vi "Settings.vi"(0 "error in":errorcluster, 1 "Channel A Settings":T2={"Enabled"=FALSE, "Coupling"=1, "Range"=6, "Analogue Offset"=0.0} {"Range" items=["10 mV", "20 mV", "50 mV", "100 mV", "200 mV", "500 mV", "1 V", "2 V", "5 V", "10 V", "20 V"]; "Coupling" items=["AC", "DC"]}, 2 "Port 0 Settings":cluster{"Enabled":bool, "Logic Level":i16}={"Enabled"=FALSE, "Logic Level"=9830} {"Logic Level" items=["1.5V TTL"=9830, "2.5V CMOS"=16383]}, 3 "Channel B Settings":T2={"Enabled"=FALSE, "Coupling"=1, "Range"=6, "Analogue Offset"=0.0} {"Range" items=["10 mV", "20 mV", "50 mV", "100 mV", "200 mV", "500 mV", "1 V", "2 V", "5 V", "10 V", "20 V"]; "Coupling" items=["AC", "DC"]}, 5 "handle in":i16, 9 "Device Info":T1, 11 "Trigger Settings":T3={"Trigger Enabled"=FALSE, "Trigger Source"=enum."Channel A", "Trigger Threshold (volts)"=0.0, "Trigger Direction"=2, "Trigger Delay (samples)"=0, "Auto Trigger Time (ms)"=1000} {"Trigger Direction" items=["Rising"=2, "Falling"=3]}, 12 "Channel C Settings":T2={"Enabled"=FALSE, "Coupling"=1, "Range"=6, "Analogue Offset"=0.0} {"Range" items=["10 mV", "20 mV", "50 mV", "100 mV", "200 mV", "500 mV", "1 V", "2 V", "5 V", "10 V", "20 V"]; "Coupling" items=["AC", "DC"]}, 13 "Port 1 Settings":cluster{"Enabled":bool, "Logic Level":i16}={"Enabled"=FALSE, "Logic Level"=9830} {"Logic Level" items=["1.5V TTL"=9830, "2.5V CMOS"=16383]}, 14 "Channel D Settings":T2={"Enabled"=FALSE, "Coupling"=1, "Range"=6, "Analogue Offset"=0.0} {"Range" items=["10 mV", "20 mV", "50 mV", "100 mV", "200 mV", "500 mV", "1 V", "2 V", "5 V", "10 V", "20 V"]; "Coupling" items=["AC", "DC"]}, 15 "Max ADC value":i16) -> (4 "error out":errorcluster, 6 "handle out":i16, 8 "enabled array":i16[](array[numeric]))   [LabVIEW 2017]
doc: "This VI is used to set up the oscilloscope. The inputs are clusters for setting channel and simple trigger settings. Advanced triggers can be set up using PicoScope3000aAdvancedTriggerSettings.vi"
uses:
  ps5000a.dll
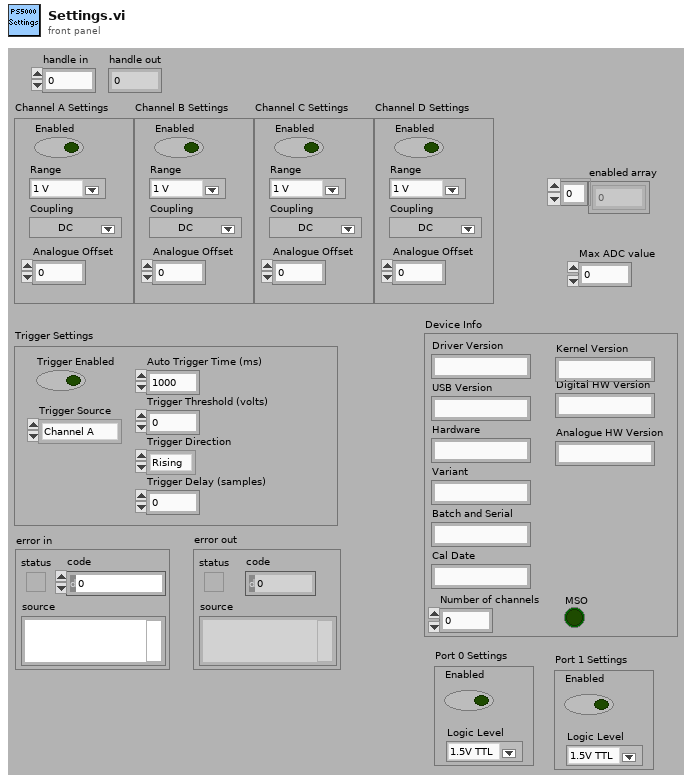
[diagram p1: front panel]
types:
  T1 = cluster{"Driver Version":string, "USB Version":string, "Hardware":string, "Variant":string, "Batch and Serial":string, "Cal Date":string, "Kernel Version":string, "Digital HW Version":string, "Analogue HW Version":string, "MSO":bool, "Number of channels":i16}
  T2 = cluster{"Enabled":bool, "Coupling":i16, "Range":u16, "Analogue Offset":sgl}
  T3 = cluster{"Trigger Enabled":bool, "Trigger Source":enum16{"Channel A", "Channel B", "Channel C", "Channel D", "Ext."}, "Trigger Threshold (volts)":dbl, "Trigger Direction":u16, "Trigger Delay (samples)":u32, "Auto Trigger Time (ms)":i16}
  T4 = enum16{"Channel A", "Channel B", "Channel C", "Channel D", "Ext."}
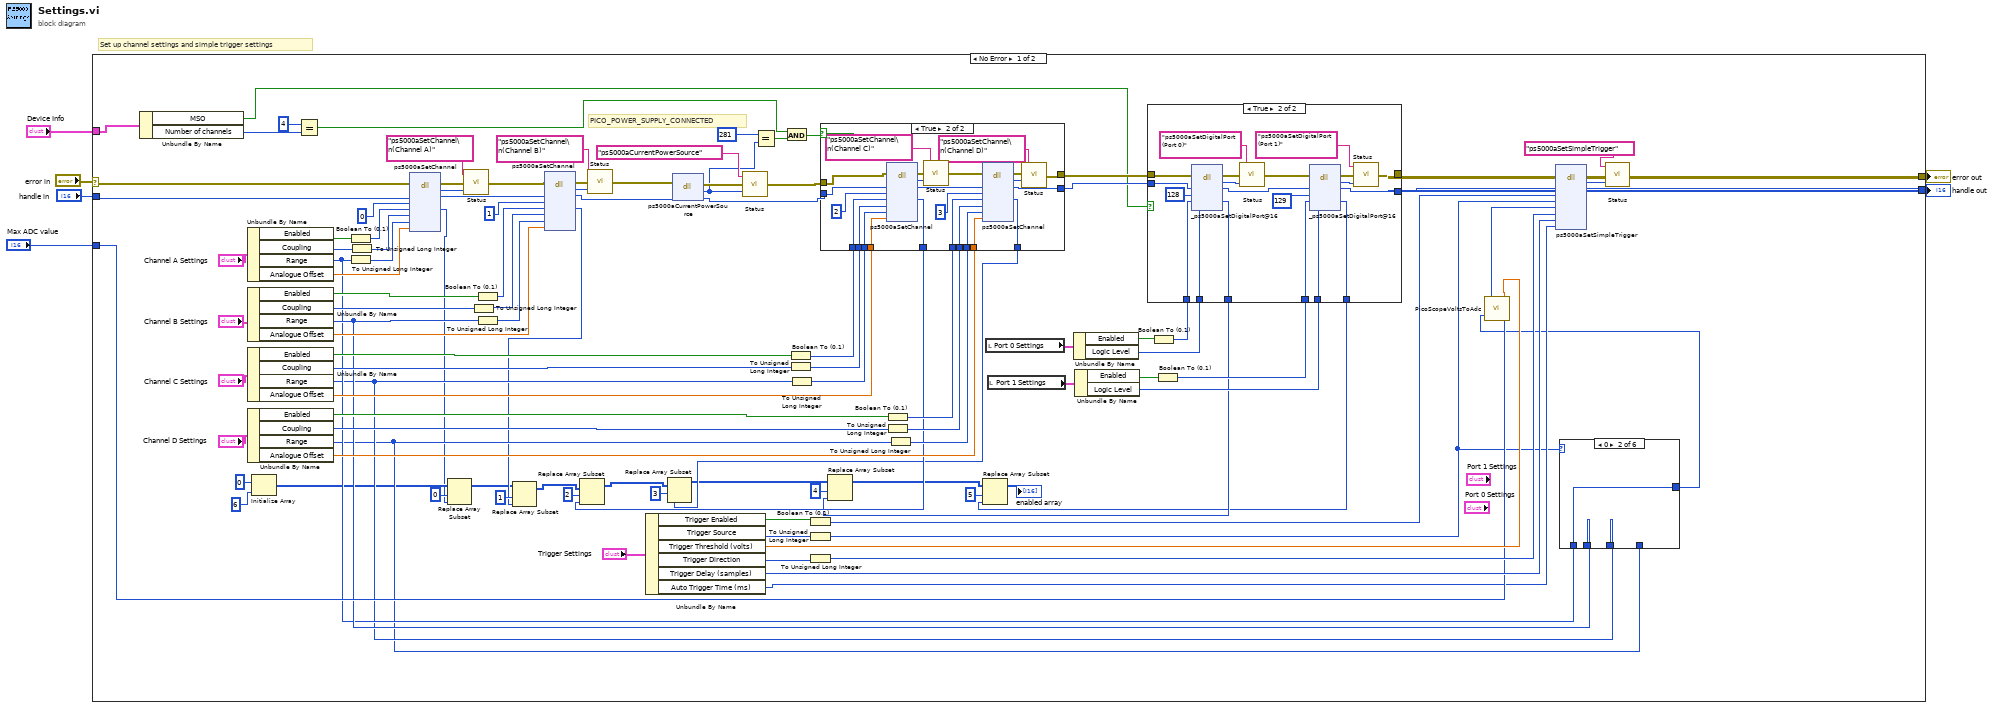
[diagram p0: block diagram]
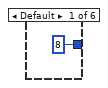
[diagram p3: hidden frame]
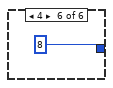
[diagram p7: hidden frame]
diagram:
  # "Set up channel settings and simple trigger settings"
  n1 = case shown="No Error" "error in" {
    selector: "error in" -> [w7 w172]
    tunnel: "handle in" -> [w35 w171]
    tunnel: [w92 w171] -> w4
    tunnel: [w47 w172] -> w3
    tunnel: "Device Info" -> [w62 _]
    tunnel: "Max ADC value" -> [w57 _]
    frame No Error {
      # "PICO_POWER_SUPPLY_CONNECTED"
      n2 = Unbundle By Name(w62) -> ("MSO"=w11:bool, "Number of channels"=w61:i16)
      n3 = Unbundle By Name("Channel A Settings") -> ("Enabled"=w104:bool, "Coupling"=w54:i16, "Range"=w51:u16, "Analogue Offset"=w87:sgl)
      n4 = Unbundle By Name("Channel B Settings") -> ("Enabled"=w103:bool, "Coupling"=w53:i16, "Range"=w52:u16, "Analogue Offset"=w81:sgl)
      n5 = Unbundle By Name("Channel C Settings") -> ("Enabled"=w102:bool, "Coupling"=w74:i16, "Range"=w50:u16, "Analogue Offset"=w79:sgl)
      n6 = Unbundle By Name("Channel D Settings") -> ("Enabled"=w101:bool, "Coupling"=w72:i16, "Range"=w49:u16, "Analogue Offset"=w78:sgl)
      n7 = Initialize Array(i16 0 ("element"), 6 ("dimension size")) -> (w31:i16[])
      n8 = Equal?(x=i16 4, y=w61) -> (x = y?=w63:bool)
      n9 = Boolean To (0,1)(Boolean=w104) -> (0, 1=w115:i16)
      n10 = To Unsigned Long Integer(number=w51) -> (unsigned 32bit integer=w88:u32)
      n11 = To Unsigned Long Integer(number=w54) -> (unsigned 32bit integer=w76:u32)
      n12 = dll-call lib="ps5000a.dll" fn="ps5000aSetChannel" ("ps3000.dll:_ps3000_open_unit@0")(error in=w7, "handle"=w35, "channel"=u32 0, "enabled"=w115, "dc"=w76, "range"=w88, "analogueOffset"=w87) -> (error out=w98:errorcluster, "PICO_STATUS"=w99:u32, "handle"=w89:i16, "enabled"=w26:i16)  [unwired: 6 in, 1 out]
      n13 = Replace Array Subset(array=w31, new element=w26, index=0) -> (w24:i16[])
      n14 = call "Status.vi"("PICO STATUS"=w99, "error in"=w98, "source"="ps5000aSetChannel\n(Channel A)") -> ("error out"=w10:errorcluster)
      n15 = To Unsigned Long Integer(number=w53) -> (unsigned 32bit integer=w77:u32)
      n16 = Boolean To (0,1)(Boolean=w103) -> (0, 1=w83:i16)
      n17 = To Unsigned Long Integer(number=w52) -> (unsigned 32bit integer=w82:u32)
      n18 = dll-call lib="ps5000a.dll" fn="ps5000aSetChannel" ("ps3000.dll:_ps3000_open_unit@0")(error in=w10, "handle"=w89, "channel"=u32 1, "enabled"=w83, "dc"=w77, "range"=w82, "analogueOffset"=w81) -> (error out=w91:errorcluster, "PICO_STATUS"=w90:u32, "handle"=w71:i16, "enabled"=w25:i16)  [unwired: 6 in, 1 out]
      n19 = Replace Array Subset(array=w24, new element=w25, index=1) -> (w23:i16[])
      n20 = call "Status.vi"("PICO STATUS"=w90, "error in"=w91, "source"="ps5000aSetChannel\n(Channel B)") -> ("error out"=w9:errorcluster)
      n21 = Unbundle By Name("Trigger Settings") -> ("Trigger Enabled"=w100:bool, "Trigger Source"=w106:T4, "Trigger Threshold (volts)"=w58:dbl, "Trigger Direction"=w108:u16, "Trigger Delay (samples)"=w107:u32, "Auto Trigger Time (ms)"=w56:i16)
      n22 = dll-call lib="ps5000a.dll" fn="ps5000aCurrentPowerSource"(error in=w9, "handle"=w71) -> (error out=w68:errorcluster, "PICO_STATUS"=w64:u32, "handle"=w66:i16)  [unwired: 2 in, 1 out]
      n23 = call "Status.vi"("PICO STATUS"=w64, "error in"=w68, "source"="ps5000aCurrentPowerSource") -> ("error out"=w67:errorcluster)
      n24 = Equal?(x=u32 281, y=w64) -> (x = y?=w34:bool)
      n25 = And(x=w63, y=w34) -> (x .and. y?=w69:bool)
      n26 = Boolean To (0,1)(Boolean=w102) -> (0, 1=w114:i16)
      n27 = To Unsigned Long Integer(number=w74) -> (unsigned 32bit integer=w75:u32)
      n28 = To Unsigned Long Integer(number=w50) -> (unsigned 32bit integer=w113:u32)
      n29 = Boolean To (0,1)(Boolean=w100) -> (0, 1=w19:i16)
      n30 = To Unsigned Long Integer(number=w106) -> (unsigned 32bit integer=w55:u32)
      n31 = To Unsigned Long Integer(number=w108) -> (unsigned 32bit integer=w110:u32)
      n32 = Boolean To (0,1)(Boolean=w101) -> (0, 1=w112:i16)
      n33 = To Unsigned Long Integer(number=w72) -> (unsigned 32bit integer=w73:u32)
      n34 = To Unsigned Long Integer(number=w49) -> (unsigned 32bit integer=w111:u32)
      n35 = case shown="True" w69 {
        tunnel: w114 -> [_ w159]
        tunnel: w113 -> [_ w157]
        tunnel: w112 -> [_ w153]
        tunnel: w111 -> [_ w152]
        tunnel: w67 -> [w146 w148]
        tunnel: [w146 w170] -> w38
        tunnel: w66 -> [w145 w163]
        tunnel: [w145 w161] -> w37
        tunnel: w75 -> [_ w158]
        tunnel: w79 -> [_ w156]
        tunnel: w73 -> [_ w155]
        tunnel: w78 -> [_ w151]
        tunnel: [_ w150] -> w21
        tunnel: [_ w149] -> w20
        frame False {
        }
        frame True {
          n36 = dll-call lib="ps5000a.dll" fn="ps5000aSetChannel" ("ps3000.dll:_ps3000_open_unit@0")(error in=w148, "handle"=w163, "channel"=u32 2, "enabled"=w159, "dc"=w158, "range"=w157, "analogueOffset"=w156) -> (error out=w167:errorcluster, "PICO_STATUS"=w166:u32, "handle"=w162:i16, "enabled"=w150:i16)  [unwired: 6 in, 1 out]
          n37 = call "Status.vi"("PICO STATUS"=w166, "error in"=w167, "source"="ps5000aSetChannel\n(Channel C)") -> ("error out"=w147:errorcluster)
          n38 = dll-call lib="ps5000a.dll" fn="ps5000aSetChannel" ("ps3000.dll:_ps3000_open_unit@0")(error in=w147, "handle"=w162, "channel"=u32 3, "enabled"=w153, "dc"=w155, "range"=w152, "analogueOffset"=w151) -> (error out=w165:errorcluster, "PICO_STATUS"=w164:u32, "handle"=w161:i16, "enabled"=w149:i16)  [unwired: 6 in, 1 out]
          n39 = call "Status.vi"("PICO STATUS"=w164, "error in"=w165, "source"="ps5000aSetChannel\n(Channel D)") -> ("error out"=w170:errorcluster)
        }
      }
      n40 = Replace Array Subset(array=w23, new element=w21, index=2) -> (w22:i16[])
      n41 = Replace Array Subset(array=w22, new element=w20, index=3) -> (w18:i16[])
      n42 = local read "Port 0 Settings"() -> (w46:cluster{"Enabled":bool, "Logic Level":i16})
      n43 = local read "Port 1 Settings"() -> (w45:cluster{"Enabled":bool, "Logic Level":i16})
      n44 = Unbundle By Name(w46) -> ("Enabled"=w44:bool, "Logic Level"=w42:i16)
      n45 = Unbundle By Name(w45) -> ("Enabled"=w41:bool, "Logic Level"=w39:i16)
      n46 = Boolean To (0,1)(Boolean=w44) -> (0, 1=w43:i16)
      n47 = Boolean To (0,1)(Boolean=w41) -> (0, 1=w40:i16)
      n48 = case shown="True" w11 {
        tunnel: [w118 w131] -> w8
        tunnel: w43 -> [_ w128]
        tunnel: w42 -> [_ w127]
        tunnel: w40 -> [_ w126]
        tunnel: w39 -> [_ w125]
        tunnel: w38 -> [w118 w120]
        tunnel: w37 -> [w117 w124]
        tunnel: [w117 w123] -> w36
        tunnel: [_ w122] -> w14
        tunnel: [_ w121] -> w13
        frame False {
        }
        frame True {
          n49 = dll-call lib="PS5000a.dll" fn="_ps5000aSetDigitalPort@16"(error in=w120, "handle"=w124, "port"=u32 128, "enabled"=w128, "logicLevel"=w127) -> (error out=w138:errorcluster, "PICO_STATUS"=w135:u32, "handle"=w132:i16, "enabled"=w122:i16)  [unwired: 4 in, 1 out]
          n50 = call "Status.vi"("PICO STATUS"=w135, "error in"=w138, "source"="ps5000aSetDigitalPort (Port 0)") -> ("error out"=w119:errorcluster)
          n51 = dll-call lib="PS5000a.dll" fn="_ps5000aSetDigitalPort@16"(error in=w119, "handle"=w132, "port"=u32 129, "enabled"=w126, "logicLevel"=w125) -> (error out=w134:errorcluster, "PICO_STATUS"=w133:u32, "handle"=w123:i16, "enabled"=w121:i16)  [unwired: 4 in, 1 out]
          n52 = call "Status.vi"("PICO STATUS"=w133, "error in"=w134, "source"="ps5000aSetDigitalPort (Port 1)") -> ("error out"=w131:errorcluster)
        }
      }
      n53 = Replace Array Subset(array=w18, new element=w14, index=4) -> (w15:i16[])
      n54 = Replace Array Subset(array=w15, new element=w13, index=5) -> (→"enabled array":i16[])
      n55 = case shown="0" w55 {
        tunnel: w51 -> [_ w140 _ _ _ _]
        tunnel: w52 -> [_ _ w141 _ _ _]
        tunnel: w50 -> [_ _ _ w142 _ _]
        tunnel: w49 -> [_ _ _ _ w143 _]
        tunnel: [u16 8 ("Range") w140 w141 w142 w143 u16 8 ("Range")] -> w48
        frame Default {
        }
        frame 0 {
        }
        frame 1 {
        }
        frame 2 {
        }
        frame 3 {
        }
        frame 4 {
        }
      }
      n56 = call "PicoScopeVoltsToAdc.vi"("Max_adc"=w57, "Volts"=w58, "Range Index"=w48) -> ("ADC count"=w59:i16)
      n57 = dll-call lib="ps5000a.dll" fn="ps5000aSetSimpleTrigger" ("ps3000.dll:_ps3000_open_unit@0")(error in=w8, "handle"=w36, "enable"=w19, "source"=w55, "threshold"=w59, "direction"=w110, "delay"=w107, "autoTrigger_ms"=w56) -> (error out=w94:errorcluster, "PICO_STATUS"=w95:u32, "handle"=w92:i16)  [unwired: 8 in, 1 out]
      n58 = call "Status.vi"("PICO STATUS"=w95, "error in"=w94, "source"="ps5000aSetSimpleTrigger") -> ("error out"=w47:errorcluster)
    }
    frame Error {
    }
  }
  "handle out" <- w4
  "error out" <- w3
